vi "Set Measure And Log Message.vi"(9 "ackNeeded":bool, 10 "args":variant, 11 "command":string) -> (3 "MyMessage":refnum<class "MeasureAndLogMessage.lvclass">)   [LabVIEW 2023, in "MeasureAndLogMessage.lvclass"]
uses:
  MeasureAndLogMessage.lvclass
  MeasureAndLogMessage.lvclass/MeasureAndLogMessage.ctl
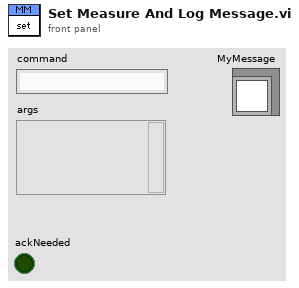
[diagram p1: front panel]
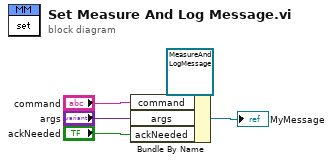
[diagram p0: block diagram]
diagram:
  n1 = Bundle By Name(cluster=refnum<class "MeasureAndLogMessage.lvclass"> refnum ("MyMessage.lvclass"), "command"="command", "args"="args", "ackNeeded"="ackNeeded") -> (→"MyMessage":refnum<class "MeasureAndLogMessage.lvclass">)
